vi "Loop_SM.vi"() -> ()   [LabVIEW 2017]
uses:
  ENUM_SM_State.ctl
  ENUM_SM_Action.ctl
  TypeDef/CLUSTER_CMD_WC_Drive.ctl
  TypeDef/ENUM_WC_Drive_DriveMode.ctl
  TypeDef/CLUSTER_Drive_ACT Loop_VBus Data.ctl
  TypeDef/CLUSTER_X and Y.ctl
  TypeDef/CLUSTER_Drive_ACT Loop_Profile Data.ctl
  TypeDef/CLUSTER_Left and Right.ctl
  TypeDef/ENUM_Drive_ACT Loop_Mode.ctl
  TypeDef/CLUSTER_Drive_HW_SRX_Status.ctl
  TypeDef/CLUSTER_4296_SRX_Status.ctl
  TypeDef/CLUSTER_SRX_Status Data.ctl
  TypeDef/CLUSTER_SRX_Encoder Data.ctl
  TypeDef/CLUSTER_SRX_PWM Data.ctl
  TypeDef/CLUSTER_SRX_Analog Data.ctl
  TypeDef/CLUSTER_SRX_Limit Switch Data.ctl
  TypeDef/CLUSTER_SRX_Profile Data.ctl
  Globals/Global_STOP.vi
  Globals/Global_CMD_Drive.vi
  Global_ACT Write_Data Out.vi
  Global_SM Write_Data Out.vi
panel:
  in  "MAX sensativity":dbl
  in  "Max RPM":dbl
  in  "MIN sensativity":dbl
  out "Cycle Time (S)":dbl format="%.3g"
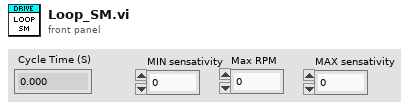
[diagram p1: front panel]
types:
  T1 = typedef "CLUSTER_Drive_HW_SRX_Status.ctl" = cluster{"Rear Left":T2, "Rear Right":T2, "Front Left":T2, "Front Right":T2}
  T2 = typedef "CLUSTER_4296_SRX_Status.ctl" = cluster{"Status":T3, "Encoder":T4, "PWM ":T5, "Analog":T6, "Limit Switches":T7, "Profile":T8}
  T3 = typedef "CLUSTER_SRX_Status Data.ctl" = cluster{"Module Enabled":bool, "Current Profile Slot Select":dbl, "Brake is Enabled":bool, "Applied Throttle":dbl, "Current":dbl, "Battery Voltage":dbl, "Sticky Fault - Under Voltage":bool, "Temperature (C)":dbl, "Sticky Fault - Over Temp":bool, "CAN Error":errorcluster, "Control 5 Is Supported":bool}
  T4 = typedef "CLUSTER_SRX_Encoder Data.ctl" = cluster{"Closed Loop Error":dbl, "Sensor Position":dbl, "Sensor Velocity":dbl, "Encoder Position":dbl, "Encoder Velocity":dbl, "Encoder Index Count":dbl, "Encoder A Pin State":bool, "Encoder B Pin State":bool, "Encoder Index Pin State":bool, "Pos Div 8":bool, "Vel Div 4":bool}
  T5 = typedef "CLUSTER_SRX_PWM Data.ctl" = cluster{"Closed Loop Error":dbl, "Pulse Width Position":i32, "Pulse Width Velocity":i32, "Pulse Width Rise To Rise (us)":i32, "Pulse Width Rise To Fall (us)":i32}
  T6 = typedef "CLUSTER_SRX_Analog Data.ctl" = cluster{"Closed Loop Error":dbl, "Analog In":dbl, "Analog In Velocity":dbl}
  T7 = typedef "CLUSTER_SRX_Limit Switch Data.ctl" = cluster{"Forward Limit Switch Closed":bool, "Reverse Limit Switch Closed":bool, "Sticky Fault - Forward Limit":bool, "Sticky Fault - Reverse Limit":bool, "Sticky Fault - Forward Soft Limit":bool, "Sticky Fault - Reverse Soft Limit":bool}
  T8 = typedef "CLUSTER_SRX_Profile Data.ctl" = cluster{"Mot Prof Active Is Under Run":bool, "Mot Prof Active Has Under Run":bool, "Mot Prof Active Is Last":bool, "Mot Prof Active Velocity Only":bool, "Mot Prof Active Is Valid":bool, "Mot Prof Buffer Is Full":bool, "Mot Prof Active Profile Slot Select":i32, "Mot Prof NextID":i32, "Mot Prof Count":i32, "Mot Prof Active Velocity":dbl, "Mot Prof Active Position":dbl, "Mot Prof Output Enable":i32}
  T9 = typedef "ENUM_Drive_ACT Loop_Mode.ctl" = enum16{"Stop", "VBus", "Profile"}
  T10 = typedef "CLUSTER_Left and Right.ctl" = cluster{"Left":dbl, "Right":dbl}
  T11 = typedef "CLUSTER_CMD_WC_Drive.ctl" = cluster{"Drive_Mode":T12, "VBus":T13, "Profile":T15}
  T12 = typedef "ENUM_WC_Drive_DriveMode.ctl" = enum16{"Motion Profile", "VBus", "Stop"}
  T13 = typedef "CLUSTER_Drive_ACT Loop_VBus Data.ctl" = cluster{"Drive":T14, "Turbo":bool}
  T14 = typedef "CLUSTER_X and Y.ctl" = cluster{"Steer":dbl, "Throtle":dbl}
  T15 = typedef "CLUSTER_Drive_ACT Loop_Profile Data.ctl" = cluster{"Start":bool}
  T16 = typedef "ENUM_SM_Action.ctl" = enum16{"No Action", "Reset Time", "Reset All", "Drive", "Shift", "Calculate Sensitivity"}
  T17 = typedef "ENUM_SM_State.ctl" = enum16{"Startup", "VBus", "Idle", "Shutdown"}
  T18 = cluster{"Action":T16, "State":T17, "Previous State":T17, "Current Time":timestamp, "Previous Time":timestamp, "Start Time":timestamp, "Target Time (ms)":u32, "Cycle Time(S)":dbl, "CMD_Drive":T11, "VBus Output":T10, "Mode Output":T9, "MQuickStopAccumulator":dbl, "SRX_Status":T1, "Sensitivity":dbl}
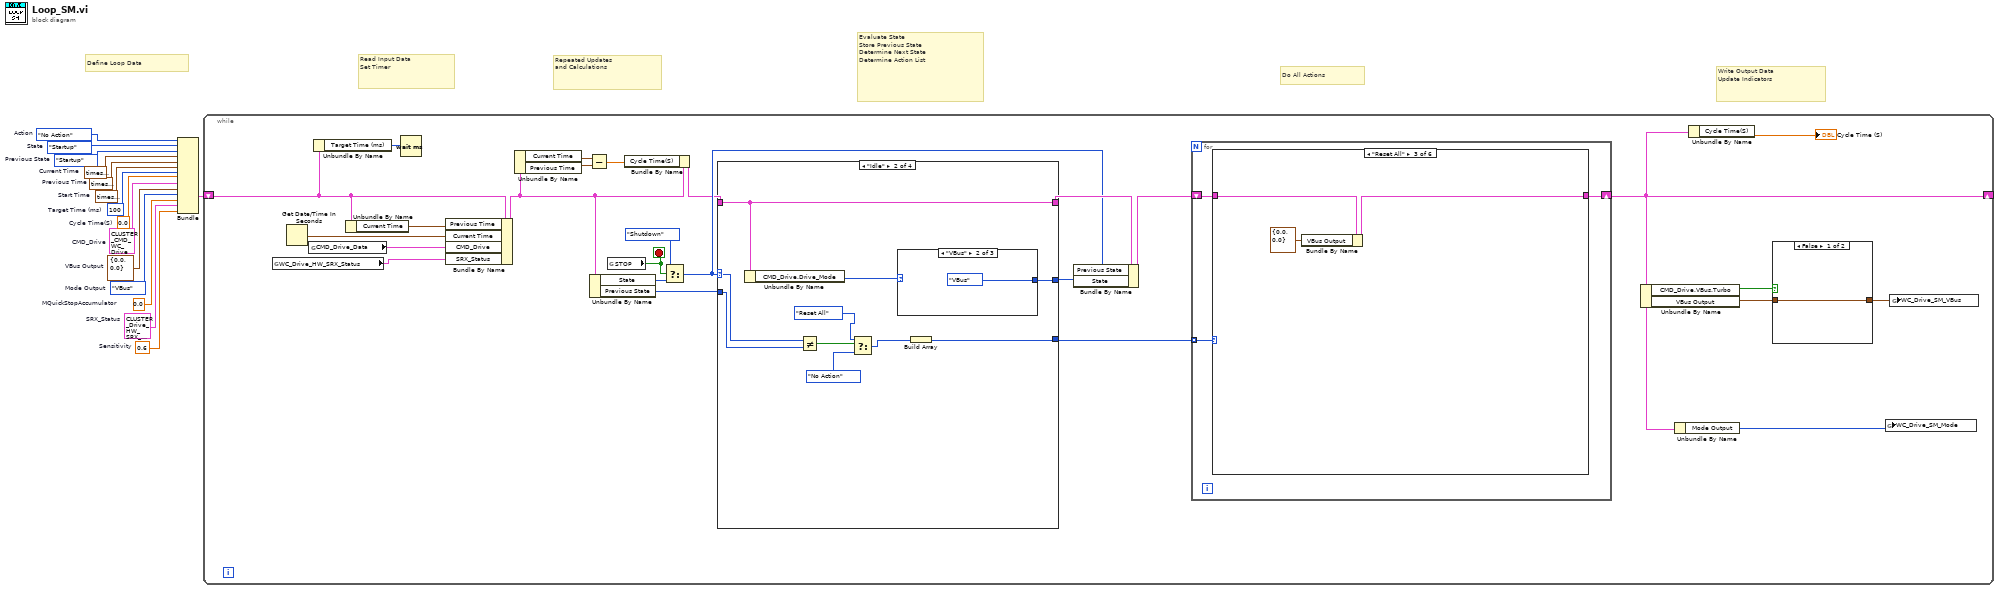
[diagram p0: block diagram]
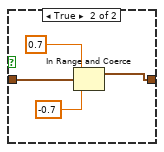
[diagram p2: hidden frame]
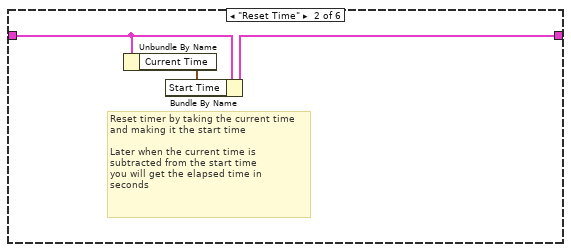
[diagram p4: hidden frame]
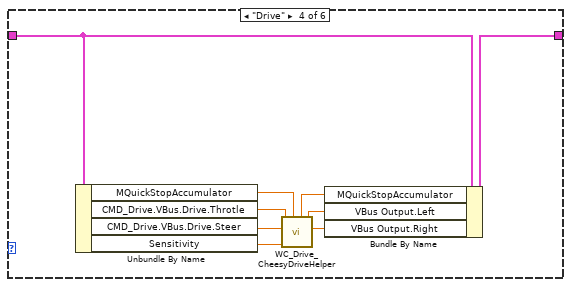
[diagram p5: hidden frame]
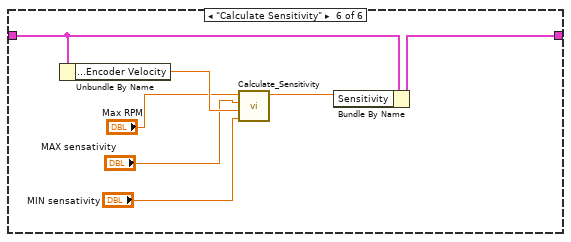
[diagram p7: hidden frame]
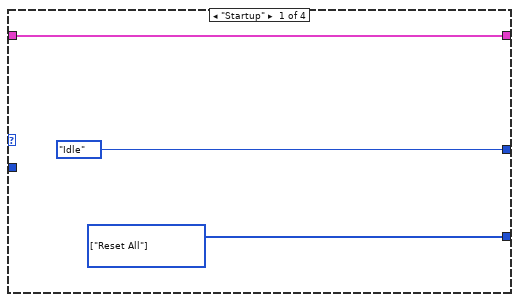
[diagram p8: hidden frame]
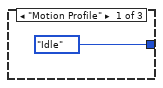
[diagram p9: hidden frame]
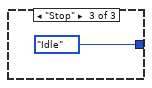
[diagram p10: hidden frame]
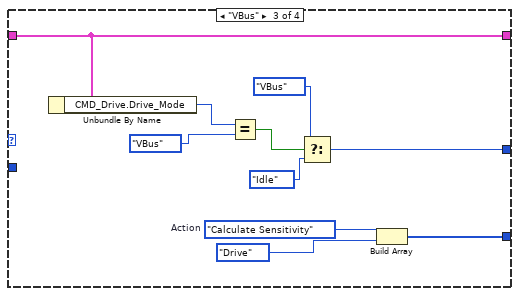
[diagram p11: hidden frame]
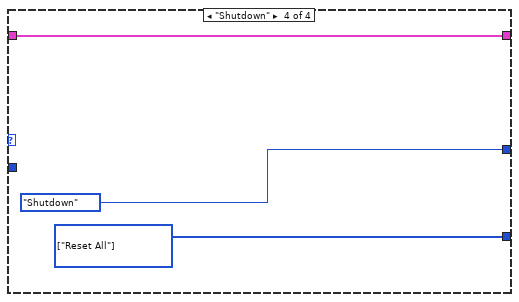
[diagram p12: hidden frame]
diagram:
  w1 = 0.6  # Sensitivity
  w2 = T1 {"Rear Left"={"Status"={"Module Enabled"=FALSE, "Current Profile Slot Select"=0.0, "Brake is Enabled"=TRUE, "Applied Throttle"=0.0, "Current"=0.0, "Battery Voltage"=12.450000000000001, "Sticky Fault - Under Voltage"=TRUE, "Temperature (C)"=30.645161290322577, "Sticky Fault - Over Temp"=FALSE, "CAN Error"={"status"=FALSE, "code"=0, "source"=""}, "Control 5 Is Supported"=TRUE}, "Encoder"={"Closed Loop Error"=0.0, "Sensor Position"=-847.859619140625, "Sensor Velocity"=0.0, "Encoder Position"=-3472833.0, "Encoder Velocity"=0.0, "Encoder Index Count"=-9452.0, "Encoder A Pin State"=FALSE, "Encoder B Pin State"=FALSE, "Encoder Index Pin State"=FALSE, "Pos Div 8"=FALSE, "Vel Div 4"=FALSE}, "PWM "={"Closed Loop Error"=0.0, "Pulse Width Position"=-3472224, "Pulse Width Velocity"=0, "Pulse Width Rise To Rise (us)"=4187, "Pulse Width Rise To Fall (us)"=1210}, "Analog"={"Closed Loop Error"=0.0, "Analog In"=105.0, "Analog In Velocity"=0.0}, "Limit Switches"={"Forward Limit Switch Closed"=FALSE, "Reverse Limit Switch Closed"=FALSE, "Sticky Fault - Forward Limit"=FALSE, "Sticky Fault - Reverse Limit"=TRUE, "Sticky Fault - Forward Soft Limit"=FALSE, "Sticky Fault - Reverse Soft Limit"=FALSE}, "Profile"={"Mot Prof Active Is Under Run"=FALSE, "Mot Prof Active Has Under Run"=FALSE, "Mot Prof Active Is Last"=FALSE, "Mot Prof Active Velocity Only"=FALSE, "Mot Prof Active Is Valid"=FALSE, "Mot Prof Buffer Is Full"=FALSE, "Mot Prof Active Profile Slot Select"=0, "Mot Prof NextID"=0, "Mot Prof Count"=0, "Mot Prof Active Velocity"=0.0, "Mot Prof Active Position"=0.0, "Mot Prof Output Enable"=0}}, "Rear Right"={"Status"={"Module Enabled"=FALSE, "Current Profile Slot Select"=0.0, "Brake is Enabled"=TRUE, "Applied Throttle"=0.0, "Current"=0.125, "Battery Voltage"=12.4, "Sticky Fault - Under Voltage"=TRUE, "Temperature (C)"=27.41935483870968, "Sticky Fault - Over Temp"=FALSE, "CAN Error"={"status"=FALSE, "code"=0, "source"=""}, "Control 5 Is Supported"=TRUE}, "Encoder"={"Closed Loop Error"=0.0, "Sensor Position"=-228.95263671875, "Sensor Velocity"=0.0, "Encoder Position"=937790.0, "Encoder Velocity"=0.0, "Encoder Index Count"=2928.0, "Encoder A Pin State"=FALSE, "Encoder B Pin State"=TRUE, "Encoder Index Pin State"=TRUE, "Pos Div 8"=FALSE, "Vel Div 4"=FALSE}, "PWM "={"Closed Loop Error"=0.0, "Pulse Width Position"=937817, "Pulse Width Velocity"=0, "Pulse Width Rise To Rise (us)"=4128, "Pulse Width Rise To Fall (us)"=3960}, "Analog"={"Closed Loop Error"=0.0, "Analog In"=103.0, "Analog In Velocity"=0.0}, "Limit Switches"={"Forward Limit Switch Closed"=FALSE, "Reverse Limit Switch Closed"=FALSE, "Sticky Fault - Forward Limit"=FALSE, "Sticky Fault - Reverse Limit"=FALSE, "Sticky Fault - Forward Soft Limit"=FALSE, "Sticky Fault - Reverse Soft Limit"=FALSE}, "Profile"={"Mot Prof Active Is Under Run"=FALSE, "Mot Prof Active Has Under Run"=FALSE, "Mot Prof Active Is Last"=FALSE, "Mot Prof Active Velocity Only"=FALSE, "Mot Prof Active Is Valid"=FALSE, "Mot Prof Buffer Is Full"=FALSE, "Mot Prof Active Profile Slot Select"=0, "Mot Prof NextID"=0, "Mot Prof Count"=0, "Mot Prof Active Velocity"=0.0, "Mot Prof Active Position"=0.0, "Mot Prof Output Enable"=0}}, "Front Left"={"Status"={"Module Enabled"=FALSE, "Current Profile Slot Select"=0.0, "Brake is Enabled"=TRUE, "Applied Throttle"=0.0, "Current"=0.0, "Battery Voltage"=12.4, "Sticky Fault - Under Voltage"=TRUE, "Temperature (C)"=28.709677419354833, "Sticky Fault - Over Temp"=FALSE, "CAN Error"={"status"=FALSE, "code"=0, "source"=""}, "Control 5 Is Supported"=TRUE}, "Encoder"={"Closed Loop Error"=0.0, "Sensor Position"=0.0, "Sensor Velocity"=0.0, "Encoder Position"=0.0, "Encoder Velocity"=0.0, "Encoder Index Count"=0.0, "Encoder A Pin State"=TRUE, "Encoder B Pin State"=TRUE, "Encoder Index Pin State"=TRUE, "Pos Div 8"=FALSE, "Vel Div 4"=FALSE}, "PWM "={"Closed Loop Error"=0.0, "Pulse Width Position"=0, "Pulse Width Velocity"=0, "Pulse Width Rise To Rise (us)"=0, "Pulse Width Rise To Fall (us)"=0}, "Analog"={"Closed Loop Error"=0.0, "Analog In"=105.0, "Analog In Velocity"=0.0}, "Limit Switches"={"Forward Limit Switch Closed"=FALSE, "Reverse Limit Switch Closed"=FALSE, "Sticky Fault - Forward Limit"=FALSE, "Sticky Fault - Reverse Limit"=FALSE, "Sticky Fault - Forward Soft Limit"=FALSE, "Sticky Fault - Reverse Soft Limit"=FALSE}, "Profile"={"Mot Prof Active Is Under Run"=FALSE, "Mot Prof Active Has Under Run"=FALSE, "Mot Prof Active Is Last"=FALSE, "Mot Prof Active Velocity Only"=FALSE, "Mot Prof Active Is Valid"=FALSE, "Mot Prof Buffer Is Full"=FALSE, "Mot Prof Active Profile Slot Select"=0, "Mot Prof NextID"=0, "Mot Prof Count"=0, "Mot Prof Active Velocity"=0.0, "Mot Prof Active Position"=0.0, "Mot Prof Output Enable"=0}}, "Front Right"={"Status"={"Module Enabled"=FALSE, "Current Profile Slot Select"=0.0, "Brake is Enabled"=TRUE, "Applied Throttle"=0.0, "Current"=0.0, "Battery Voltage"=12.35, "Sticky Fault - Under Voltage"=TRUE, "Temperature (C)"=26.77419354838709, "Sticky Fault - Over Temp"=FALSE, "CAN Error"={"status"=FALSE, "code"=0, "source"=""}, "Control 5 Is Supported"=TRUE}, "Encoder"={"Closed Loop Error"=0.0, "Sensor Position"=0.0, "Sensor Velocity"=0.0, "Encoder Position"=0.0, "Encoder Velocity"=0.0, "Encoder Index Count"=0.0, "Encoder A Pin State"=TRUE, "Encoder B Pin State"=TRUE, "Encoder Index Pin State"=TRUE, "Pos Div 8"=FALSE, "Vel Div 4"=FALSE}, "PWM "={"Closed Loop Error"=0.0, "Pulse Width Position"=0, "Pulse Width Velocity"=0, "Pulse Width Rise To Rise (us)"=0, "Pulse Width Rise To Fall (us)"=0}, "Analog"={"Closed Loop Error"=0.0, "Analog In"=102.0, "Analog In Velocity"=0.0}, "Limit Switches"={"Forward Limit Switch Closed"=FALSE, "Reverse Limit Switch Closed"=FALSE, "Sticky Fault - Forward Limit"=FALSE, "Sticky Fault - Reverse Limit"=TRUE, "Sticky Fault - Forward Soft Limit"=FALSE, "Sticky Fault - Reverse Soft Limit"=FALSE}, "Profile"={"Mot Prof Active Is Under Run"=FALSE, "Mot Prof Active Has Under Run"=FALSE, "Mot Prof Active Is Last"=FALSE, "Mot Prof Active Velocity Only"=FALSE, "Mot Prof Active Is Valid"=FALSE, "Mot Prof Buffer Is Full"=FALSE, "Mot Prof Active Profile Slot Select"=0, "Mot Prof NextID"=0, "Mot Prof Count"=0, "Mot Prof Active Velocity"=0.0, "Mot Prof Active Position"=0.0, "Mot Prof Output Enable"=0}}}  # SRX_Status
  w3 = 0.0  # MQuickStopAccumulator
  w4 = ENUM_Drive_ACT_Loop_Mode."VBus"  # Mode Output
  w5 = T10 {"Left"=0.0, "Right"=0.0}  # VBus Output
  w6 = T11 {"Drive_Mode"=enum."Motion Profile", "VBus"={"Drive"={"Steer"=0.0, "Throtle"=0.0}, "Turbo"=FALSE}, "Profile"={"Start"=FALSE}}  # CMD_Drive
  w7 = ENUM_SM_Action."No Action"  # Action
  w8 = 0.0  # Cycle Time(S)
  w9 = ENUM_SM_State."Startup"  # Previous State
  w10 = timestamp(0 s since 1904-01-01)  # Previous Time
  w11 = u32 100  # Target Time (ms)
  w12 = timestamp(0 s since 1904-01-01)  # Start Time
  w13 = timestamp(0 s since 1904-01-01)  # Current Time
  w14 = ENUM_SM_State."Startup"  # State
  # "Define Loop Data"
  # "Repeated Updates\nand Calculations"
  # "Read Input Data\nSet Timer"
  # "Evaluate State\nStore Previous State\nDetermine Next State\nDetermine Action List"
  # "Do All Actions"
  # "Write Output Data\nUpdate Indicators"
  n1 = Bundle("Action"=w7, "State"=w14, "Previous State"=w9, "Current Time"=w13, "Previous Time"=w10, "Start Time"=w12, "Target Time (ms)"=w11, "Cycle Time(S)"=w8, "CMD_Drive"=w6, "VBus Output"=w5, "Mode Output"=w4, "MQuickStopAccumulator"=w3, "SRX_Status"=w2, "Sensitivity"=w1) -> (w15:T18)  [unwired: 1 in]
  n2 = while {
    shift-right: [w20] -> _
    shift-left: w15 -> [w32]
    stop <- w37 stop-if-true
    n3 = global read "Global_ACT Write_Data Out.vi" "WC_Drive_HW_SRX_Status"() -> (w16:T1)
    n4 = Get Date/Time In Seconds() -> (seconds since 1Jan1904=w41:timestamp)
    n5 = global read "Global_CMD_Drive.vi" "CMD_Drive_Data"() -> (w21:T11)
    n6 = Unbundle By Name(w32) -> ("Target Time (ms)"=w34:u32)
    n7 = Unbundle By Name(w32) -> ("Current Time"=w33:timestamp)
    n8 = Wait (ms)(milliseconds to wait=w34) -> ()  [unwired: 1 out]
    n9 = Bundle By Name(cluster=w32, "Previous Time"=w33, "Current Time"=w41, "CMD_Drive"=w21, "SRX_Status"=w16) -> (w26:T18)
    n10 = Unbundle By Name(w26) -> ("Current Time"=w27:timestamp, "Previous Time"=w28:timestamp)
    n11 = Subtract(x=w27, y=w28) -> (x-y=w24:dbl)
    n12 = Unbundle By Name(w26) -> ("State"=w35:T17, "Previous State"=w31:T17)
    n13 = global read "Global_STOP.vi" "STOP"() -> (w37:bool)
    n14 = Bundle By Name(cluster=w26, "Cycle Time(S)"=w24) -> (w25:T18)
    n15 = Select(t=ENUM_SM_State."Shutdown" ("State"), s=w37, f=w35) -> (s? t:f=w30:T17)
    n16 = case shown="\"Idle\"" w30 {
      selector: w30 -> [_ w80 _ _]
      tunnel: w25 -> [w76 w86 w99 w102]
      tunnel: [w76 w86 w99 w102] -> w39
      tunnel: [ENUM_SM_State."Idle" ("State") w77 w98 ENUM_SM_State."Shutdown" ("State")] -> w38
      tunnel: [w75 w81 w92 w100] -> w23
      tunnel: w31 -> [_ w79 _ _]
      frame "Startup" {
        w75 = T16[] [enum."Reset All"] items=["No Action", "Reset Time", "Reset All", "Drive", "Shift", "Calculate Sensitivity"] ("Actions")
      }
      frame "Idle" {
        n17 = Unbundle By Name(w86) -> ("CMD_Drive.Drive_Mode"=w78:T12)
        n18 = Not Equal?(x=w80, y=w79) -> (x != y?=w85:bool)
        n19 = Select(t=ENUM_SM_Action."Reset All" ("Action"), s=w85, f=ENUM_SM_Action."No Action" ("Action")) -> (s? t:f=w84:T16)
        n20 = case shown="\"VBus\"" w78 {
          tunnel: [ENUM_SM_State."Idle" ("State") ENUM_SM_State."VBus" ("State") ENUM_SM_State."Idle" ("State")] -> w77
          frame "Motion Profile" {
          }
          frame "VBus" {
          }
          frame "Stop" {
          }
        }
        n21 = Build Array(w84) -> (w81:T16[])
      }
      frame "VBus" {
        w93 = ENUM_SM_Action."Calculate Sensitivity"  # Action
        n22 = Unbundle By Name(w99) -> ("CMD_Drive.Drive_Mode"=w97:T12)
        n23 = Equal?(x=w97, y=ENUM_WC_Drive_DriveMode."VBus" ("CMD_Drive_Mode")) -> (x = y?=w96:bool)
        n24 = Select(t=ENUM_SM_State."VBus" ("State"), s=w96, f=ENUM_SM_State."Idle" ("State")) -> (s? t:f=w98:T17)
        n25 = Build Array(w93, ENUM_SM_Action."Drive" ("element")) -> (w92:T16[])
      }
      frame "Shutdown" {
        w100 = T16[] [enum."Reset All"] items=["No Action", "Reset Time", "Reset All", "Drive", "Shift", "Calculate Sensitivity"] ("Actions")
      }
    }
    n26 = Bundle By Name(cluster=w39, "Previous State"=w30, "State"=w38) -> (w40:T18)
    n27 = for {
      tunnel: w23 -> [w49] mode=indexing
      shift-right: [w48] -> w20
      shift-left: w40 -> [w47]
      n28 = case shown="\"Reset All\"" w49 {
        tunnel: w47 -> [w50 w53 w56 w65 w66 w73]
        tunnel: [w50 w52 w55 w64 w66 w72] -> w48
        frame "No Action" {
        }
        frame "Reset Time" {
          # "Reset timer by taking the current time\nand making it the start time\n\nLater when the current time is \nsubtracted from the start time\nyou will get the elapsed time in \nseconds"
          n29 = Unbundle By Name(w53) -> ("Current Time"=w51:timestamp)
          n30 = Bundle By Name(cluster=w53, "Start Time"=w51) -> (w52:T18)
        }
        frame "Reset All" {
          n31 = Bundle By Name(cluster=w56, "VBus Output"=T10 {"Left"=0.0, "Right"=0.0}) -> (w55:T18)
        }
        frame "Drive" {
          n32 = Unbundle By Name(w65) -> ("MQuickStopAccumulator"=w62:dbl, "CMD_Drive.VBus.Drive.Throtle"=w61:dbl, "CMD_Drive.VBus.Drive.Steer"=w60:dbl, "Sensitivity"=w59:dbl)
          n33 = call "WC_Drive_CheesyDriveHelper.vi"("MQuickStopAccumulator"=w62, "KTurnSensitivity"=w59, "Steer"=w60, "Throttle"=w61) -> ("RightPwm Out"=w57:dbl, "LeftPwm Out"=w58:dbl, "MQuickStopAccumulator Out"=w63:dbl)  [unwired: 5 in]
          n34 = Bundle By Name(cluster=w65, "MQuickStopAccumulator"=w63, "VBus Output.Left"=w58, "VBus Output.Right"=w57) -> (w64:T18)
        }
        frame "Shift" {
        }
        frame "Calculate Sensitivity" {
          n35 = Unbundle By Name(w73) -> ("SRX_Status.Rear Right.Encoder.Encoder Velocity"=w70:dbl)
          n36 = call "Calculate_Sensitivity.vi"("Min Sensitivity"="MIN sensativity", "Current RPM"=w70, "Max Sensitivity"="MAX sensativity", "Max RPM"="Max RPM") -> ("Sensitivity"=w71:dbl)  [unwired: 7 in]
          n37 = Bundle By Name(cluster=w73, "Sensitivity"=w71) -> (w72:T18)
        }
      }
    }
    n38 = Unbundle By Name(w20) -> ("CMD_Drive.VBus.Turbo"=w17:bool, "VBus Output"=w22:T10)
    n39 = Unbundle By Name(w20) -> ("Mode Output"=w19:T9)
    n40 = Unbundle By Name(w20) -> ("Cycle Time(S)"=→"Cycle Time (S)":dbl)
    n41 = case shown="False" w17 {
      tunnel: w22 -> [w42 w46]
      tunnel: [w42 w43] -> w18
      frame False {
      }
      frame True {
        n42 = In Range and Coerce(upper limit=0.7, x=w46, lower limit=-0.7) -> (coerced(x)=w43:T10)  [unwired: 1 out]
      }
    }
    n43 = global write "Global_SM Write_Data Out.vi" "WC_Drive_SM_Mode"(w19) -> ()
    n44 = global write "Global_SM Write_Data Out.vi" "WC_Drive_SM_VBus"(w18) -> ()
  }
